vi "Paste FP from CLipboard.vi"(8 "error in":errorcluster, 10 "Write/Read Cell":T1={"Cell Range"="", "Data 2D"=[], "Select Sheet"="", "1 Data"="", "Data 1D"=[], "Font col"=0, "Bold"=TRUE, "Font Size"=18, "Inside lines"=FALSE}, 11 "Work Sheet 2":refnum<k7>) -> (0 "error out":errorcluster, 3 "Work Sheet":refnum<k7>)   [LabVIEW 2017]
uses:
  controls/read.write.ctl
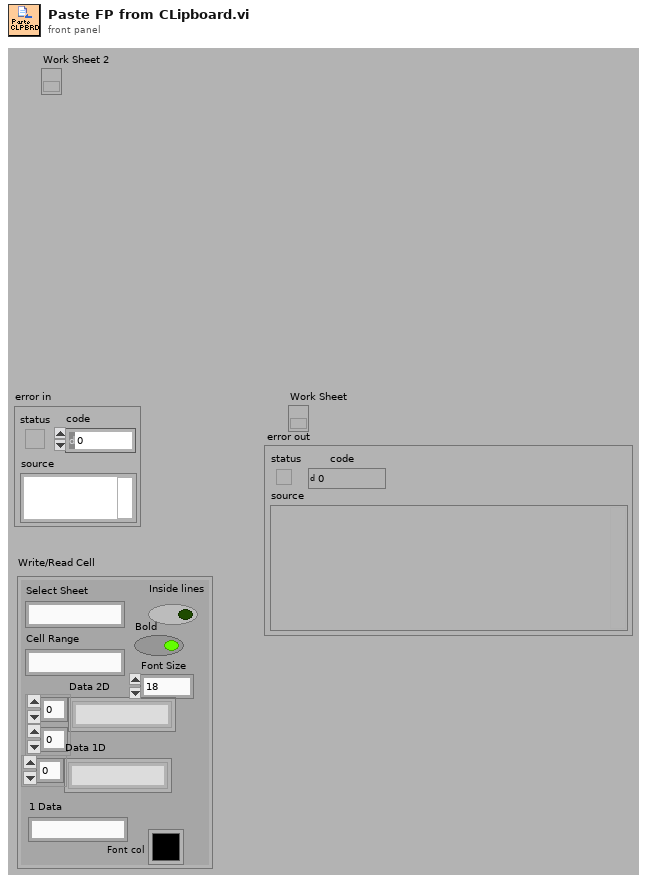
[diagram p1: front panel]
types:
  T1 = typedef "read.write.ctl" = cluster{"Cell Range":string, "Data 2D":string[][], "Select Sheet":string, "1 Data":string, "Data 1D":string[], "Font col":u32, "Bold":bool, "Font Size":i32, "Inside lines":bool}
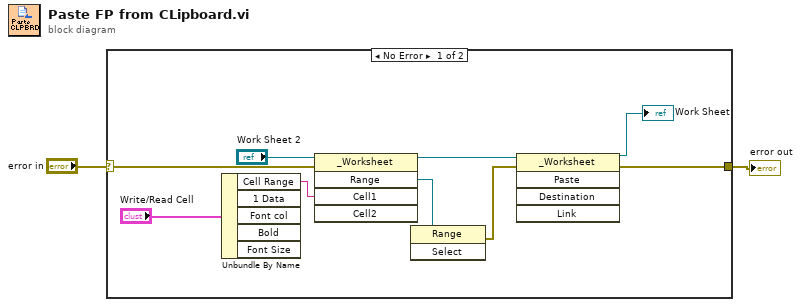
[diagram p0: block diagram]
diagram:
  n1 = case shown="No Error" "error in" {
    selector: "error in" -> [w8 w12]
    tunnel: [w3 w12] -> w1
    frame No Error {
      n2 = Unbundle By Name("Write/Read Cell") -> ("Cell Range"=w9:string)  [unwired: 4 out]
      n3 = invoke class="_Worksheet" method="Range"(reference="Work Sheet 2", error in=w8, "Cell1"=w9) -> (reference out=w4:refnum<k7>, "Range"=w6:refnum<k7>)  [unwired: 2 in, 3 out]
      n4 = invoke class="Range" method="Select"(reference=w6) -> (error out=w5:errorcluster)  [unwired: 2 in, 2 out]
      n5 = invoke class="_Worksheet" method="Paste"(reference=w4, error in=w5) -> (reference out=→"Work Sheet":refnum<k7>, error out=w3:errorcluster)  [unwired: 3 in, 3 out]
    }
    frame Error {
    }
  }
  "error out" <- w1
